vi "Drive System.vi"(9 "Buttons":T1, 10 "Axes":T2) -> ()   [LabVIEW 2012]
uses:
  <vilib>/Rock Robotics/WPI/Joystick/WPI_JoystickButtonState.ctl
  <vilib>/Rock Robotics/WPI/Solenoid/WPI_SolenoidValue.ctl
  <vilib>/addons/control/pid/pid.llb/PID Control Input Filter (DBL).vi
  <vilib>/Rock Robotics/WPI/Solenoid/WPI_SolenoidSetEnum.vi
  <vilib>/Rock Robotics/WPI/RobotDrive/WPI_RobotDriveGetSetRefNum.vi
  <vilib>/addons/control/pid/NI_PID_pid.lvlib
panel:
  out "PID X":dbl(graph)
  out "X":dbl(graph)
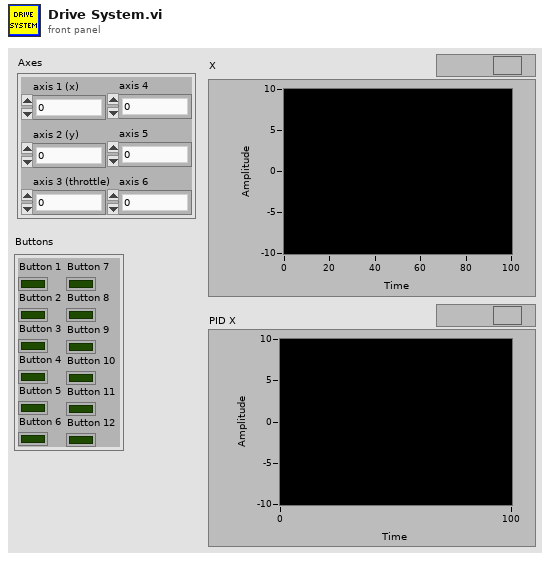
[diagram p1: front panel]
types:
  T1 = typedef "WPI_JoystickButtonState.ctl" = cluster{"Button 1":bool, "Button 2":bool, "Button 3":bool, "Button 4":bool, "Button 5":bool, "Button 6":bool, "Button 7":bool, "Button 8":bool, "Button 9":bool, "Button 10":bool, "Button 11":bool, "Button 12":bool}
  T2 = cluster{"axis 1 (x)":dbl, "axis 2 (y)":dbl, "axis 3 (throttle)":dbl, "axis 4":dbl, "axis 5":dbl, "axis 6":dbl}
  T3 = typedef "WPI_SolenoidValue.ctl" = enum16{"Off", "On", "Forward", "Reverse"}
  T4 = typedef "WPI_SolenoidDevRef.ctl" = cluster{"DevStatus":errorcluster, "Solenoid Module":T5, "Forward Solenoid Channel":T6, "Reverse Solenoid Channel":T6}
  T5 = typedef "FPGA_TypedefSolenoidModule.ctl" = enum16{"Solenoid Module 1", "Solenoid Module 2"}
  T6 = typedef "WPI_SolenoidChannel.ctl" = enum8{"Solenoid 1", "Solenoid 2", "Solenoid 3", "Solenoid 4", "Solenoid 5", "Solenoid 6", "Solenoid 7", "Solenoid 8", "Invalid"}
  T7 = typedef "WPI_RobotDriveDevRef.ctl" = cluster{"DevStatus":errorcluster, "Motors[]":T8[], "Square Inputs":bool, "Max Output":dbl, "Isochronous":bool}
  T8 = typedef "WPI_MotorControlDeviceRef.ctl" = cluster{"DeviceStatus":errorcluster, "Type":enum16{"PWM", "CAN"}, "PWM":cluster{"Digital Module":T9, "PWM Channel":T10, "DeadBand":T11}, "CAN":cluster{"Device Number":u8, "Control Mode":T12, "Semaphore":T13, "Max Vout":dbl}, "Invert":bool, "TransformRef":T14, "InvTransformRef":T14}
  T9 = typedef "FPGA_TypedefDigitalModule.ctl" = enum16{"Digital Module 1", "Digital Module 2"}
  T10 = typedef "FPGA_DIOPWMChannel.ctl" = enum8{"PWM 1", "PWM 2", "PWM 3", "PWM 4", "PWM 5", "PWM 6", "PWM 7", "PWM 8", "PWM 9", "PWM 10", "Invalid"}
  T11 = typedef "WPI_PWMDeadband.ctl" = cluster{"Name":string, "maxPositivePwm":i32, "minPositivePwm":i32, "centerPwm":i32, "maxNegativePwm":i32, "minNegativePwm":i32, "angularRange":u16}
  T12 = typedef "WPI_CANJaguar_ControlMode.ctl" = enum8{"Percent VBus", "Current", "Speed", "Position", "Voltage"}
  T13 = typedef "Semaphore RefNum" = refnum<k1>
  T14 = typedef "WPI_PWMTransform_ConPane.ctl" = refnum<vi>
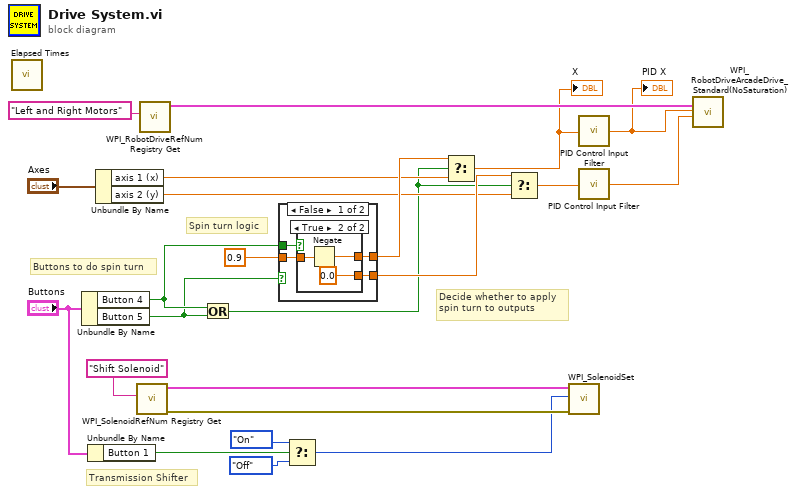
[diagram p0: block diagram]
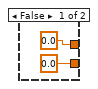
[diagram p2: hidden frame]
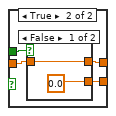
[diagram p3: hidden frame]
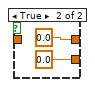
[diagram p4: hidden frame]
diagram:
  # "Transmission Shifter"
  # "Spin turn logic"
  # "Buttons to do spin turn"
  # "Decide whether to apply\nspin turn to outputs"
  n1 = call "Elapsed Times.vi"() -> ()  [unwired: 3 in, 1 out]
  n2 = Unbundle By Name("Buttons") -> ("Button 4"=w21:bool, "Button 5"=w18:bool)
  n3 = Unbundle By Name("Buttons") -> ("Button 1"=w5:bool)
  n4 = Unbundle By Name("Axes") -> ("axis 1 (x)"=w10:dbl, "axis 2 (y)"=w9:dbl)
  n5 = call <vilib>:"WPI_SolenoidRefNum Registry Get.vi"("refnum name"="Shift Solenoid") -> ("error out"=w3:errorcluster, "SolenoidDevRef"=w4:T4)  [unwired: 9 in]
  n6 = call <vilib>:"WPI_RobotDriveRefNum Registry Get.vi"("refnum name"="Left and Right Motors") -> ("RobotDriveDevRef"=w23:T7)  [unwired: 1 in, 9 out]
  n7 = Or(x=w21, y=w18) -> (x .or. y?=w2:bool)
  n8 = case shown="False" w18 {
    tunnel: w21 -> [w27 w34]
    tunnel: [w26 w36] -> w20
    tunnel: [w25 w35] -> w19
    tunnel: 0.9 -> [w24 w33]
    frame False {
      n9 = case shown="True" w27 {
        tunnel: [0.0 w31] -> w26
        tunnel: [0.0 0.0] -> w25
        tunnel: w24 -> [_ w30]
        frame False {
        }
        frame True {
          n10 = Negate(x=w30) -> (-x=w31:dbl)
        }
      }
    }
    frame True {
      n11 = case shown="False" w34 {
        tunnel: [w37 0.0] -> w36
        tunnel: [0.0 0.0] -> w35
        tunnel: w33 -> [w37 _]
        frame False {
        }
        frame True {
        }
      }
    }
  }
  n12 = Select(t=WPI_SolenoidValue."On" ("Value"), s=w5, f=WPI_SolenoidValue."Off" ("Value")) -> (s? t:f=w1:T3)
  n13 = Select(t=w20, s=w2, f=w10) -> (s? t:f=w15:dbl)
  "X" <- w15
  n14 = Select(t=w19, s=w2, f=w9) -> (s? t:f=w14:dbl)
  n15 = call-poly <vilib>:"WPI_SolenoidSet.vi"("error in (no error)"=w3, "Value"=w1, "SolenoidDevRef"=w4) -> ()  [unwired: 7 in, 2 out]
  n16 = call-poly <vilib>:"PID Control Input Filter.vi"("input"=w15) -> ("output"=w11:dbl)  [unwired: 4 in]
  "PID X" <- w11
  n17 = call-poly <vilib>:"PID Control Input Filter.vi"("input"=w14) -> ("output"=w13:dbl)  [unwired: 4 in]
  n18 = call <vilib>:"WPI_RobotDriveArcadeDrive_Standard(NoSaturation).vi"("Y axis value"=w13, "X axis value"=w11, "RobotDriveDevRef"=w23) -> ()  [unwired: 1 in, 8 out]
